vi "Simulation.vi"() -> ()   [LabVIEW 2013]
doc: "This VI starts and stops the environment simulator and serves as the master VI for your simulation code. Open and run this VI to display the environment simulator, or open the block diagram to view or modify simulation code."
uses:
  <vilib>/robotics/Simulator/Engine/ctl/DeviceID.ctl
  <instrlib>/Hokuyo URG Series/HAIOL/Hokuyo URG Series.lvclass
  <vilib>/robotics/Simulator/NI_Robotics_Simulator.lvlib
  <instrlib>/Hokuyo URG Series/HAIOL/Simulator/Hokuyo URG Series Simulator.lvclass
panel:
  out "XY Graph":cluster{dbl[], dbl[]}(graph)
  out "3D Picture":refnum<vi>(3d-picture)
  in  "stop":bool
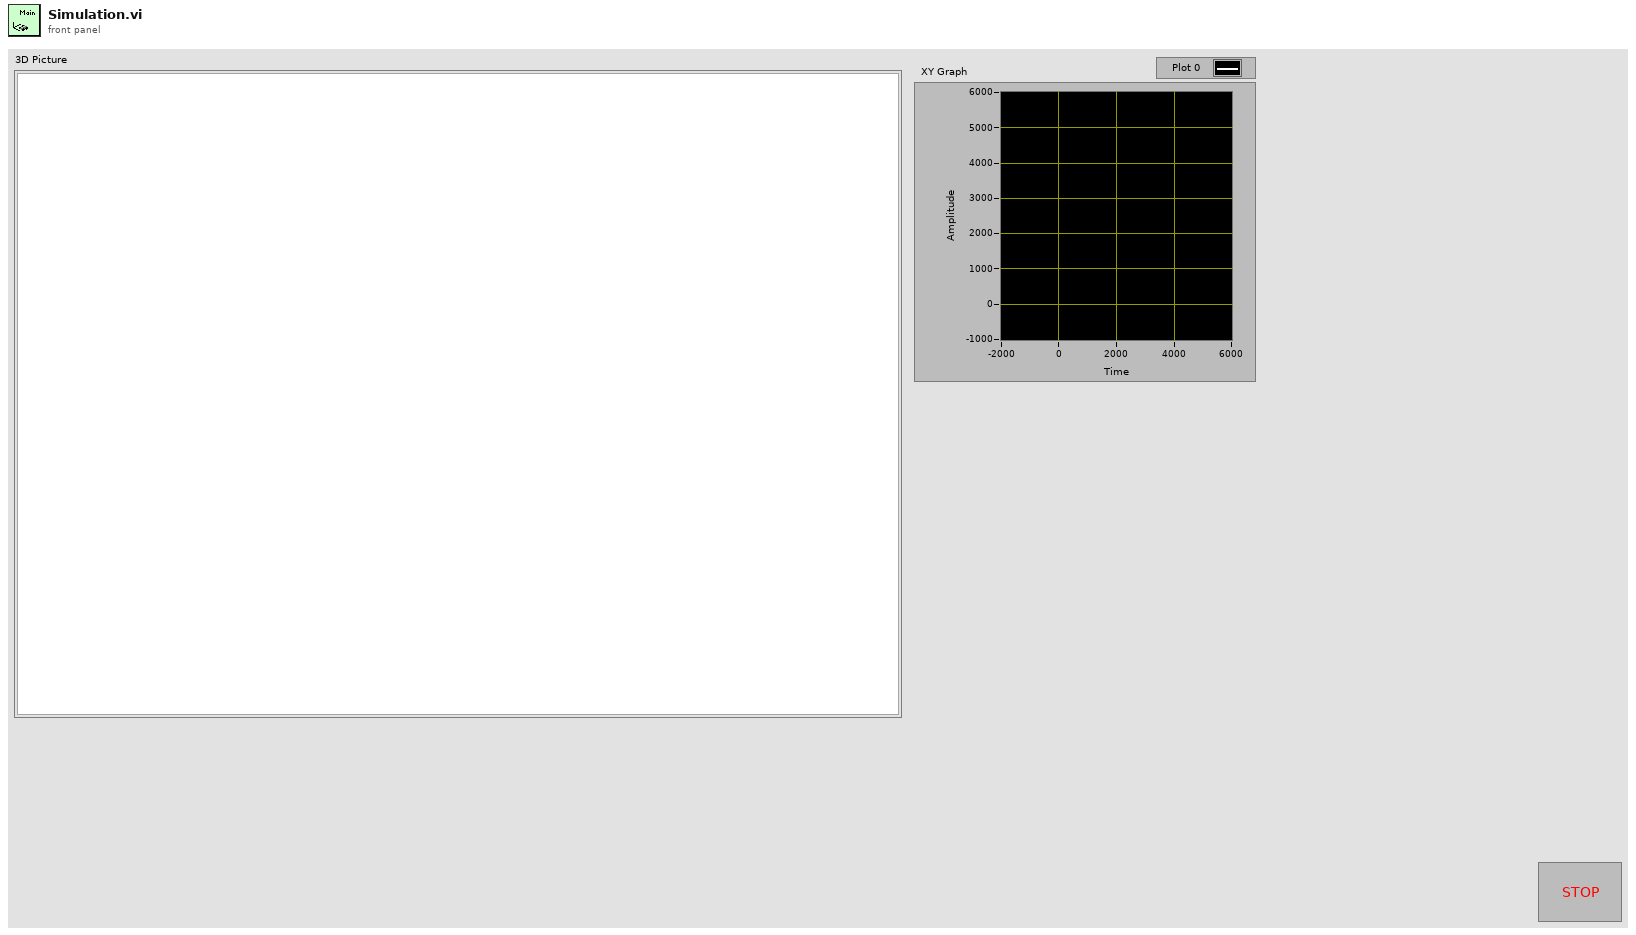
[diagram p1: front panel]
types:
  T1 = typedef "NI_Robotics_Simulator.lvlib/DeviceID.ctl" = cluster{"robot ID":string, "sensor/actuator ID":string}
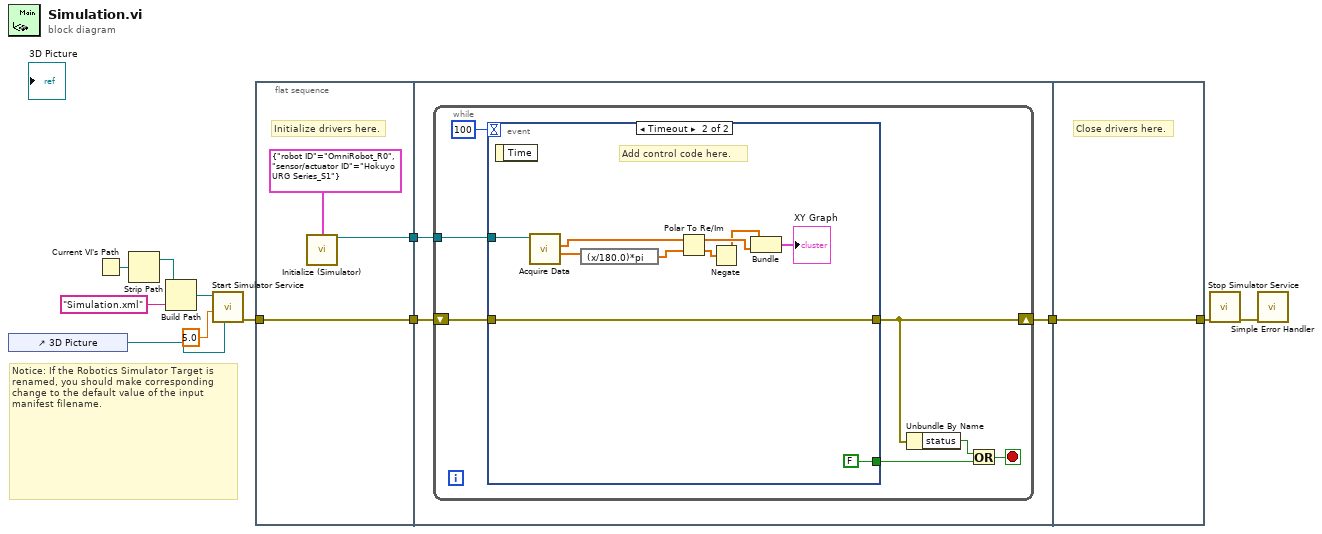
[diagram p0: block diagram]
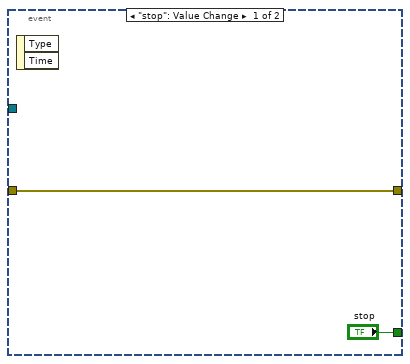
[diagram p2: hidden frame]
diagram:
  # "Notice: If the Robotics Simulator Target is renamed, you should make corresponding change to the default value of the input manifest filename."
  n1 = control-ref of="3D Picture"() -> (w2:refnum<vi>)
  n2 = Current VI's Path() -> (path=w10:path)
  n3 = Strip Path(path=w10) -> (stripped path=w9:path)  [unwired: 1 out]
  n4 = Build Path(base path=w9, name or relative path="Simulation.xml" ("manifest filename")) -> (appended path=w8:path)
  n5 = call <vilib>:"Start Simulator Service.vi"("3D picture refnum"=w2, "step size (ms)"=5.0 ("stepsize(ms)"), "manifest file"=w8) -> ("error out"=w6:errorcluster)  [unwired: 8 in]
  n6 = flat-sequence {
    tunnel: w6 -> [w15]
    tunnel: [w15] -> w5
    tunnel: [w13] -> w1
    tunnel: w5 -> [w17]
    tunnel: [w18] -> w4
    tunnel: w1 -> [w16]
    tunnel: [w38] -> w11
    tunnel: w4 -> [w38]
    frame #0 {
      # "Initialize drivers here."
      n7 = call <instrlib>:"Initialize (Simulator).vi"("Device ID"=T1 {"robot ID"="OmniRobot_R0", "sensor/actuator ID"="Hokuyo URG Series_S1"}) -> ("Hokuyo URG Series out"=w13:refnum<class "Hokuyo URG Series.lvclass">)  [unwired: 13 in, 1 out]
    }
    frame #1 {
      n8 = while {
        shift-right: [w21] -> w18
        shift-left: w17 -> [w24]
        tunnel: w16 -> [w19]
        stop <- w22 stop-if-true
        n9 = event shown="[1] Timeout" {
          selector: _ -> [_ _]
          dyn-events: _ -> [_ _]
          timeout: 100 -> [_ _]
          tunnel: ["stop" FALSE ("stop")] -> w23
          tunnel: [w26 w37] -> w21
          tunnel: w24 -> [w26 w37]
          tunnel: w19 -> [_ w35]
          event "stop": Value Change {
            n10 = event-data() -> ()  [unwired: 1 in, 2 out]
          }
          event Timeout {
            # "Add control code here."
            n11 = event-data() -> ()  [unwired: 1 in, 1 out]
            n12 = call-dynamic "Acquire Data.vi"("Hokuyo URG Series in"=w35) -> ("Direction"=w34:dbl[], "Magnitude"=w33:dbl[])  [unwired: 7 in, 2 out]
            n13 = expression code="(x/180.0)*pi" ("degrees to radians")(w34) -> (w32:dbl[])
            n14 = Polar To Re/Im(2:w32, 3:w33) -> (0:w30:dbl[], 1:w29:dbl[])
            n15 = Negate(x=w30) -> (-x=w28:dbl[])
            n16 = Bundle(w28, w29) -> (→"XY Graph":cluster{dbl[], dbl[]})  [unwired: 1 in]
          }
        }
        n17 = Unbundle By Name(w21) -> ("status"=w20:bool)
        n18 = Or(x=w20, y=w23) -> (x .or. y?=w22:bool)
      }
    }
    frame #2 {
      # "Close drivers here."
    }
  }
  n19 = call <vilib>:"Stop Simulator Service.vi"("error in (no error)"=w11) -> ("error out"=w7:errorcluster)  [unwired: 10 in]
  n20 = call <vilib>:"Simple Error Handler.vi"("error in (no error)"=w7) -> ()  [unwired: 4 in, 5 out]
